vi "Add.vi"(10 "y":dbl, 11 "x":dbl) -> (2 "x+y":dbl)   [LabVIEW 2019]
panel:
  in  "Waveform":waveform(dbl)
  out "Waveform Graph":dbl[](graph)
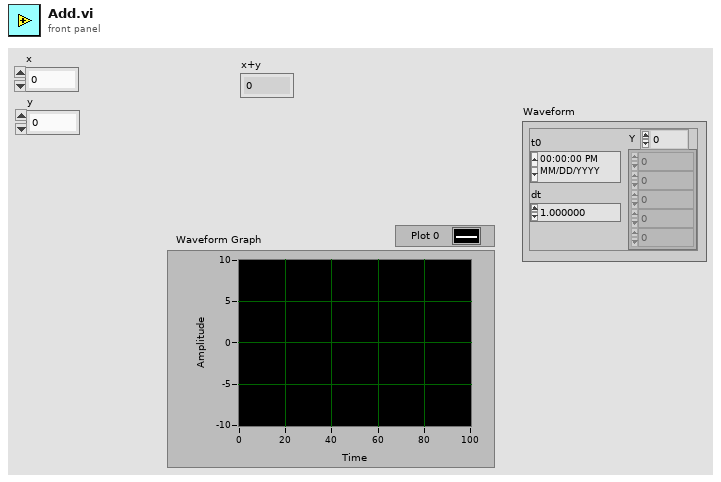
[diagram p1: front panel]
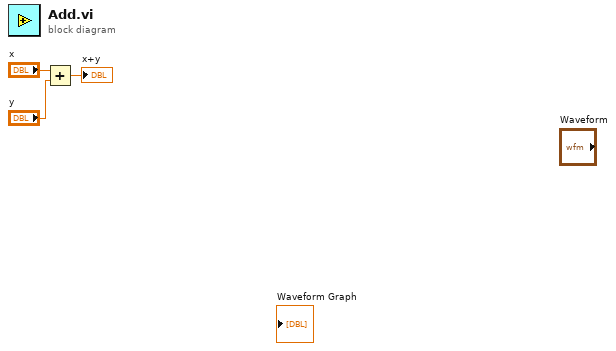
[diagram p0: block diagram]
diagram:
  n1 = Add(x="x", y="y") -> (x+y=→"x+y":dbl)
